vi "radius_neighbors_graph.vi"(8 "error in (no error)":errorcluster caption="entrée d'erreur (pas d'erreur)", 11 "RNeighbors.lvclass":refnum<class "RNeighbors.lvclass">) -> (0 "error out":errorcluster caption="sortie d'erreur", 2 "A":dbl[][](array[numeric]), 3 "RNeighbors.lvclass 2":refnum<class "RNeighbors.lvclass">)   [LabVIEW 2020, in "RNeighbors.lvclass"]
doc: "Computes the (weighted) graph of Neighbors for points in X\n\nNeighborhoods are restricted the points at a distance lower than radius.\n\nParameters\nX : array-like of shape (n_samples, n_features), default=None\nThe query point or points. If not provided, neighbors of each indexed point are returned. In this case, the query point is not considered its own neighbor.\n\nradius : float, default=None\nRadius of neighborhoods. The default is the value passed to the constructor.\n\nmode : {‘connectivity’, ‘distance’}, default=’connectivity’\nType of returned matrix: ‘connectivity’ will return the connectivity matrix with ones and zeros, in ‘distance’ the edges are Euclidean distance between points.\n\nsort_results : bool, default=False\nIf True, in each row of the result, the non-zero entries will be sorted by increasing distances. If False, the non-zero entries may not be sorted. Only used with mode=’distance’."
uses:
  RNeighbors.lvclass
  C:/Users/cipop/TDF Dropbox/2_Technologies de France/1 - Services et Etudes/PLAIY/2 - DEV/PLAIYLAB/code/Python/Python.lvclass
  C:/Users/cipop/TDF Dropbox/2_Technologies de France/1 - Services et Etudes/PLAIY/2 - DEV/PLAIYLAB/code/Model/Model.lvclass
  C:/Users/cipop/TDF Dropbox/2_Technologies de France/1 - Services et Etudes/PLAIY/2 - DEV/PLAIYLAB/code/Model/Supervised/Neighbors/Neighbors.lvclass
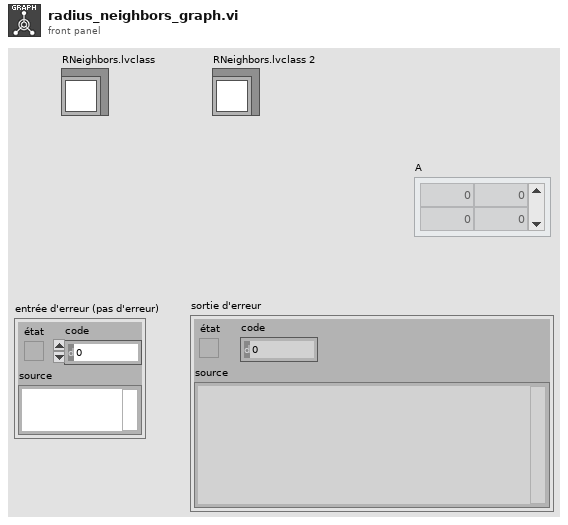
[diagram p1: front panel]
types:
  T1 = typedef "data.ctl" = cluster{"name":string, "X":dbl[][]}
  T2 = typedef "neighbors_data.ctl" = cluster{"y":dbl[][], "sample_weight":dbl[]}
  T3 = typedef "rneighbors_data.ctl" = cluster{"radius":dbl, "mode":string, "return_distance":bool, "sort_results":bool}
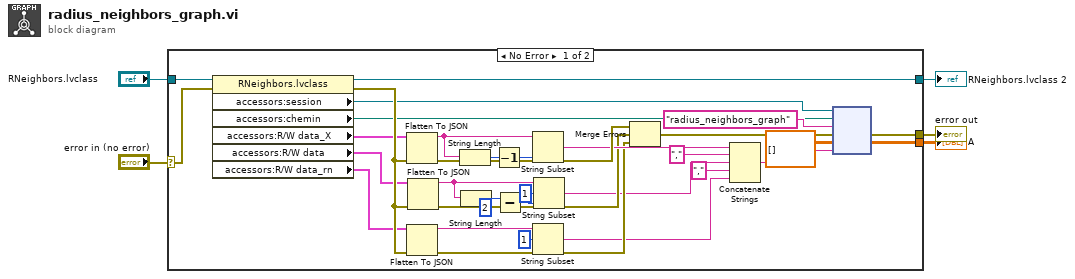
[diagram p0: block diagram]
diagram:
  n1 = case shown="No Error" "error in (no error)" {
    selector: "error in (no error)" -> [w36 w40]
    tunnel: [w37 w40] -> w2
    tunnel: [w8 w39] -> w3
    tunnel: "RNeighbors.lvclass" -> [w35 w39]
    tunnel: [w6 _] -> w1
    frame No Error {
      n2 = property class="RNeighbors.lvclass"(reference=w35, error in=w36) -> (reference out=w8:refnum<class "RNeighbors.lvclass">, error out=w24:errorcluster, "accessors:session"=w11:refnum<k35>, "accessors:chemin"=w10:path, "accessors:R/W data_X"=w13:T1, "accessors:R/W data"=w12:T2, "accessors:R/W data_rn"=w16:T3)
      n3 = Flatten To JSON(anything=w13, error in (no error)=w24) -> (JSON string=w32:string, 11:w29:errorcluster)  [unwired: 1 in]
      n4 = Flatten To JSON(anything=w16, error in (no error)=w24) -> (JSON string=w30:string, 11:w22:errorcluster)  [unwired: 1 in]
      n5 = Flatten To JSON(anything=w12, error in (no error)=w24) -> (JSON string=w20:string, 11:w21:errorcluster)  [unwired: 1 in]
      n6 = String Length(string=w32) -> (length=w34:i32)
      n7 = String Length(string=w20) -> (length=w15:i32)
      n8 = Decrement(x=w34) -> (x-1=w33:i32)
      n9 = Subtract(x=w15, y=2) -> (x-y=w25:i32)
      n10 = String Subset(string=w32, length (rest)=w33) -> (substring=w27:string)  [unwired: 1 in]
      n11 = String Subset(string=w30, offset (0)=1) -> (substring=w17:string)  [unwired: 1 in]
      n12 = String Subset(string=w20, offset (0)=1, length (rest)=w25) -> (substring=w19:string)
      n13 = Merge Errors(w29, w21, w22) -> (w9:errorcluster)
      n14 = Concatenate Strings(w27, "," ("string"), w19, "," ("string"), w17) -> (w26:string)
      n15 = node(w11, w10, "radius_neighbors_graph" ("nom de la fonction"), w9, dbl[][] [] ("A"), w26) -> (w37:errorcluster, w6:dbl[][])  [unwired: 1 in, 3 out]
    }
    frame Error {
    }
  }
  "error out" <- w2
  "RNeighbors.lvclass 2" <- w3
  "A" <- w1
